vi "Check Coefficients.vi"(0 "CalChannelsDisplay":string[][](array[string]), 2 "New Data":bool, 5 "Checkbox Array":bool[](array[boolean]), 7 "TrackingRowsSel":i32[](array[numeric]), 9 "AllCoeffIndexes In":i32[](array[numeric])) -> (8 "AllCoeffIndexes Out":i32[](array[numeric]), 10 "CurrentCoeffIndexes Out":i32[](array[numeric]), 15 "Enable Apply":bool)   [LabVIEW 2013]
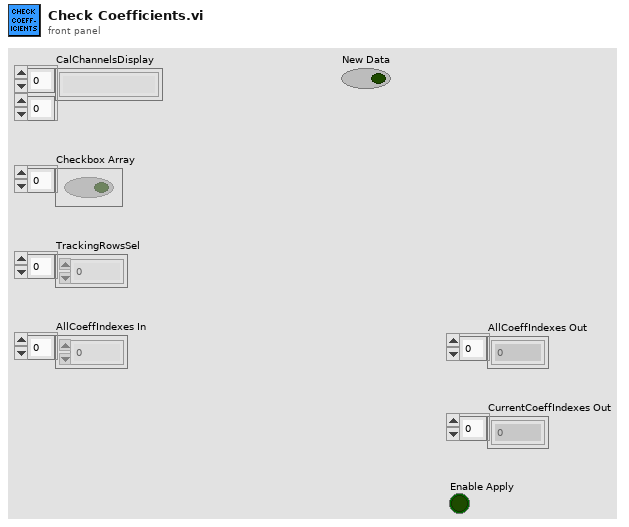
[diagram p1: front panel]
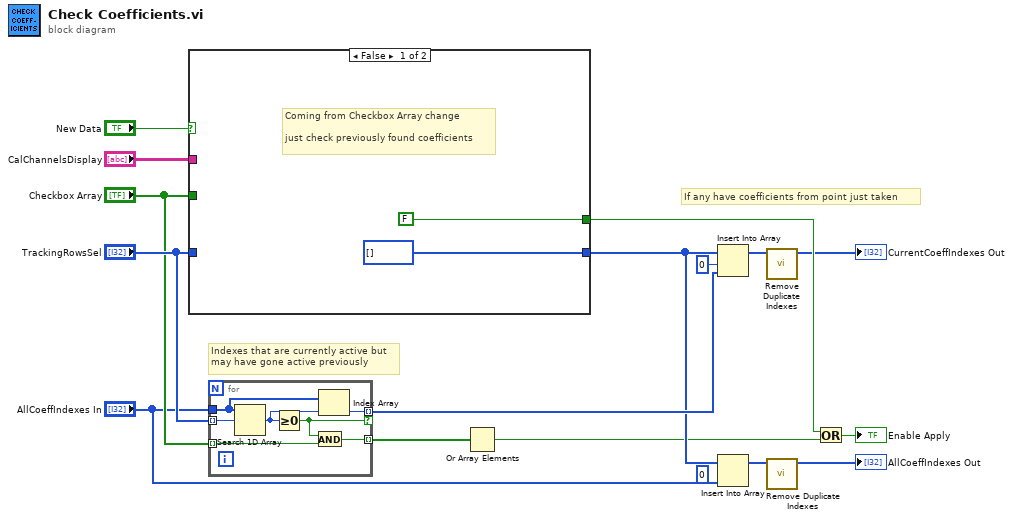
[diagram p0: block diagram]
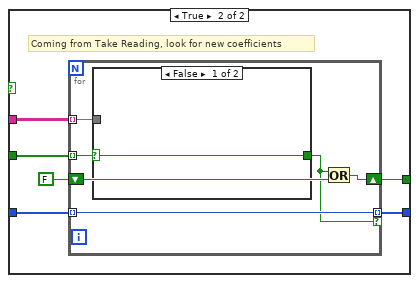
[diagram p2: hidden frame]
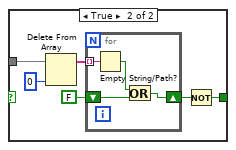
[diagram p3: hidden frame]
diagram:
  (unwired) 0 ("index")
  # "Indexes that are currently active but\nmay have gone active previously"
  # "If any have coefficients from point just taken"
  n1 = case shown="False" "New Data" {
    tunnel: "CalChannelsDisplay" -> [_ w23]
    tunnel: "TrackingRowsSel" -> [_ w22]
    tunnel: "Checkbox Array" -> [_ w21]
    tunnel: [FALSE w20] -> w13
    tunnel: [i32[] [] w19] -> w7
    frame False {
      # "Coming from Checkbox Array change\n\njust check previously found coefficients"
    }
    frame True {
      # "Coming from Take Reading, look for new coefficients"
      n2 = for {
        tunnel: w23 -> [w30] mode=indexing
        tunnel: w21 -> [w29] mode=indexing
        shift-right: [w27] -> w20
        shift-left: FALSE -> [w28]
        tunnel: [w26] -> w19 mode=indexing if=w25
        tunnel: w22 -> [w26] mode=indexing
        n3 = case shown="False" w29 {
          selector: w29 -> [w31 _]
          tunnel: w30 -> [_ w37]
          tunnel: [w31 w32] -> w25
          frame False {
          }
          frame True {
            n4 = Delete From Array(array=w37, index=0) -> (array with subset deleted=w35:string[])  [unwired: 1 in, 1 out]
            n5 = for {
              tunnel: w35 -> [w41] mode=indexing
              shift-right: [w38] -> w33
              shift-left: FALSE -> [w40]
              n6 = Empty String/Path?(string/path=w41) -> (empty?=w39:bool)
              n7 = Or(x=w39, y=w40) -> (x .or. y?=w38:bool)
            }
            n8 = Not(x=w33) -> (.not. x?=w32:bool)
          }
        }
        n9 = Or(x=w25, y=w28) -> (x .or. y?=w27:bool)
      }
    }
  }
  n10 = for {
    tunnel: "AllCoeffIndexes In" -> [w44]
    tunnel: "TrackingRowsSel" -> [w48] mode=indexing
    tunnel: [w42] -> w10 mode=indexing if=w46
    tunnel: "Checkbox Array" -> [w47] mode=indexing
    tunnel: [w45] -> w3 mode=indexing
    n11 = Search 1D Array(1D array=w44, element=w48) -> (index of element=w43:i32)  [unwired: 1 in]
    n12 = Greater Or Equal To 0?(x=w43) -> (x >= 0?=w46:bool)
    n13 = And(x=w46, y=w47) -> (x .and. y?=w45:bool)
    n14 = Index Array(array=w44, index=w43) -> (element=w42:i32)
  }
  n15 = Or Array Elements(Boolean array=w3) -> (logical OR=w2:bool)
  n16 = Insert Into Array(array=w7, index=0, new element=w10) -> (w9:i32[])
  n17 = Insert Into Array(array=w7, new element="AllCoeffIndexes In") -> (w5:i32[])  [unwired: 1 in]
  n18 = call "Remove Duplicate Indexes.vi"("Indexes In"=w9) -> ("Indexes Out"=→"CurrentCoeffIndexes Out":i32[])  [unwired: 10 in]
  n19 = call "Remove Duplicate Indexes.vi"("Indexes In"=w5) -> ("Indexes Out"=→"AllCoeffIndexes Out":i32[])  [unwired: 10 in]
  n20 = Or(x=w13, y=w2) -> (x .or. y?=→"Enable Apply":bool)
